vi "FT_Read_Byte_Data.vi"(10 "Bytes To Read":u32, 11 "Handle":u32) -> (0 "error out":errorcluster, 1 "FT_Status":u32(ring) items=["FT_OK", "FT_INVALID_HANDLE", "FT_DEVICE_NOT_FOUND", "FT_DEVICE_NOT_OPENED", "FT_IO_ERROR", "FT_INSUFFICIENT_RESOURCES", "FT_INVALID_PARAMETER", "FT_INVALID_BAUD_RATE", "FT_DEVICE_NOT_OPENED_FOR_ERASE", "FT_DEVICE_NOT_OPENED_FOR_WRITE", "FT_FAILED_TO_WRITE_DEVICE", "FT_EEPROM_READ_FAILED", "FT_EEPROM_WRITE_FAILED", "FT_EEPROM_ERASE_FAILED", "FT_EEPROM_NOT_PRESENT", "FT_EEPROM_NOT_PROGRAMMED", "FT_INVALID_ARGS", "FT_NOT_SUPPORTED", "FT_OTHER_ERROR"], 2 "Bytes Read":u32, 3 "Read Data":u8[](array[numeric]))   [LabVIEW 2011]
uses:
  ftd2xx.dll
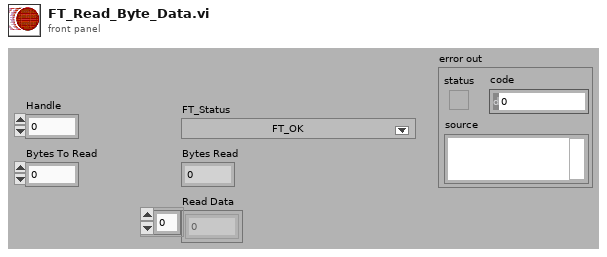
[diagram p1: front panel]
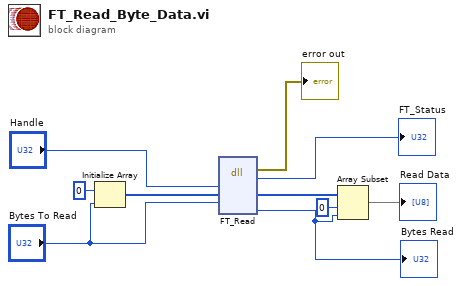
[diagram p0: block diagram]
diagram:
  n1 = Initialize Array(u8 0 ("element"), "Bytes To Read") -> (w8:u8[])
  n2 = dll-call lib="C:/Users/INL Students/Desktop/INL labview repository/3rd Party/D2XX_Functions_7.0/FTD2XX.dll" fn="FT_Read"("Handle"="Handle", "Buffer"=w8, "BytesToRead"="Bytes To Read") -> (error out=→"error out":errorcluster, "FT_Status"=→"FT_Status":u32, "Buffer"=w5:u8[], "BytesReturned"=w3:u32)  [unwired: 6 in, 1 out]
  "Bytes Read" <- w3
  n3 = Array Subset(array=w5, index=0, length=w3) -> (→"Read Data":u8[])
